vi "Check_Block_Has_Landed.vi"(8 "Block":T1 {"orientaion" items=["up", "down", "left", "right"]; "type" items=["t", "rl", "ll", "rz", "lz", "square", "line"]}, 10 "Input Array":bool[][](array[boolean])) -> (0 "landed":bool)   [LabVIEW 2015]
uses:
  block.ctl
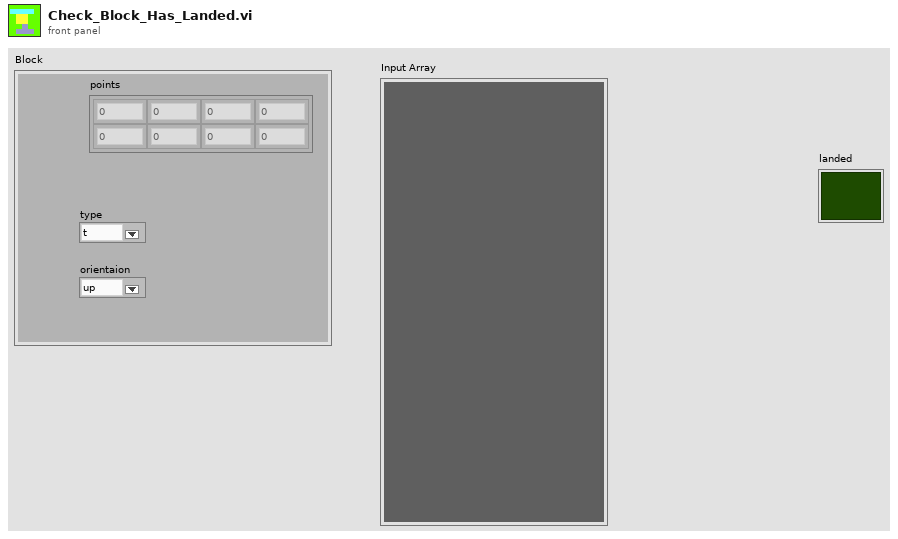
[diagram p1: front panel]
types:
  T1 = typedef "block.ctl" = cluster{"points":dbl[][], "type":u16, "orientaion":u16}
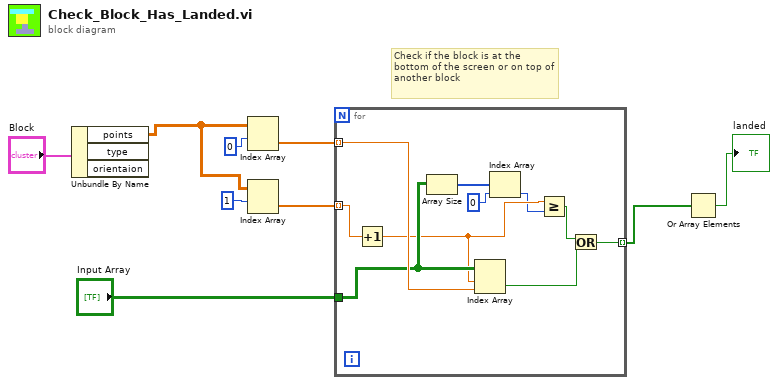
[diagram p0: block diagram]
diagram:
  # "Check if the block is at the bottom of the screen or on top of another block"
  n1 = Unbundle By Name("Block") -> ("points"=w7:dbl[][])  [unwired: 2 out]
  n2 = Index Array(array=w7, index (row)=0) -> (element=w4:dbl[])  [unwired: 1 in]
  n3 = Index Array(array=w7, index (row)=1) -> (element=w5:dbl[])  [unwired: 1 in]
  n4 = for {
    tunnel: w5 -> [w19] mode=indexing
    tunnel: w4 -> [w18] mode=indexing
    tunnel: "Input Array" -> [w17]
    tunnel: [w12] -> w1 mode=indexing
    n5 = Increment(x=w19) -> (x+1=w11:dbl)
    n6 = Array Size(array=w17) -> (size(s)=w16:i32[])
    n7 = Index Array(array=w17, index (row)=w11, index (col)=w18) -> (element=w14:bool)
    n8 = Index Array(array=w16, index=0) -> (element=w10:i32)
    n9 = Greater Or Equal?(x=w11, y=w10) -> (x >= y?=w13:bool)
    n10 = Or(x=w13, y=w14) -> (x .or. y?=w12:bool)
  }
  n11 = Or Array Elements(Boolean array=w1) -> (logical OR=→"landed":bool)
